vi "Align control label.vi"(8 "error in (no error)":errorcluster, 9 "label Position":T1, 11 "Ctl Refnum":refnum<vi>) -> (0 "error out":errorcluster, 3 "Ctl Refnum":refnum<vi>)   [LabVIEW 2009]
uses:
  label position.ctl
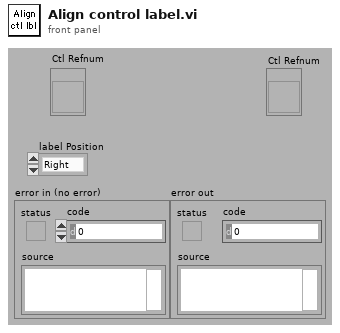
[diagram p1: front panel]
types:
  T1 = typedef "label position.ctl" = enum16{"Right", "Left", "Top left", "Top right"}
  T2 = typedef "LVPositionTypeDef.ctl" = cluster{"Left":i32, "Top":i32}
  T3 = typedef "LVBoundsTypeDef.ctl" = cluster{"Width":u32, "Height":u32}
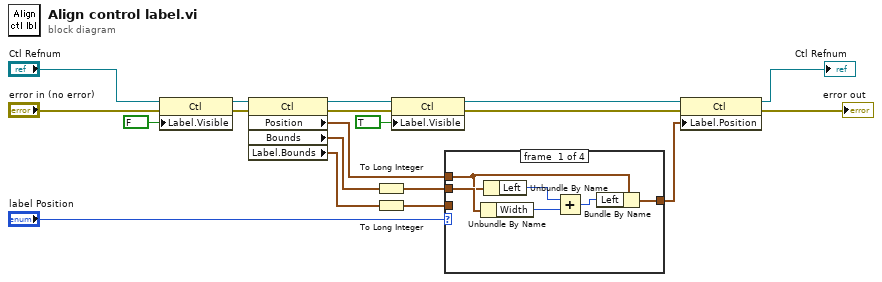
[diagram p0: block diagram]
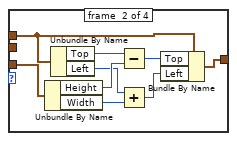
[diagram p2: hidden frame]
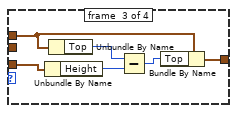
[diagram p3: hidden frame]
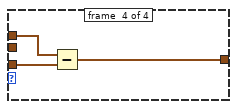
[diagram p4: hidden frame]
diagram:
  n1 = property class="Ctl"(reference="Ctl Refnum", error in="error in (no error)", "Label.Visible"=FALSE) -> (reference out=w9:refnum<vi>, error out=w7:errorcluster)
  n2 = property class="Ctl"(reference=w9, error in=w7) -> (reference out=w4:refnum<vi>, error out=w5:errorcluster, "Position"=w13:T2, "Bounds"=w14:T3, "Label.Bounds"=w18:T3)
  n3 = To Long Integer(number=w14) -> (32bit integer=w16:cluster{"Width":i32, "Height":i32})
  n4 = To Long Integer(number=w18) -> (32bit integer=w15:cluster{"Width":i32, "Height":i32})
  n5 = property class="Ctl"(reference=w4, error in=w5, "Label.Visible"=TRUE) -> (reference out=w1:refnum<vi>, error out=w2:errorcluster)
  n6 = case shown="\"Top right\"" "label Position" {
    tunnel: w16 -> [w25 _ _ _]
    tunnel: w13 -> [w23 w31 w37 w43]
    tunnel: w15 -> [_ w34 w40 w42]
    tunnel: [w22 w29 w35 w41] -> w17
    frame #0 {
      n7 = Unbundle By Name(w25) -> ("Width"=w20:i32)
      n8 = Unbundle By Name(w23) -> ("Left"=w24:i32)
      n9 = Add(x=w24, y=w20) -> (x+y=w21:i32)
      n10 = Bundle By Name(cluster=w23, "Left"=w21) -> (w22:T2)
    }
    frame #1 {
      n11 = Unbundle By Name(w34) -> ("Height"=w32:i32, "Width"=w28:i32)
      n12 = Unbundle By Name(w31) -> ("Top"=w33:i32, "Left"=w27:i32)
      n13 = Subtract(x=w33, y=w32) -> (x-y=w30:i32)
      n14 = Add(x=w27, y=w28) -> (x+y=w26:i32)
      n15 = Bundle By Name(cluster=w31, "Top"=w30, "Left"=w26) -> (w29:T2)
    }
    frame #2 {
      n16 = Unbundle By Name(w40) -> ("Height"=w38:i32)
      n17 = Unbundle By Name(w37) -> ("Top"=w39:i32)
      n18 = Subtract(x=w39, y=w38) -> (x-y=w36:i32)
      n19 = Bundle By Name(cluster=w37, "Top"=w36) -> (w35:T2)
    }
    frame #3 {
      n20 = Subtract(x=w43, y=w42) -> (x-y=w41:T2)
    }
  }
  n21 = property class="Ctl"(reference=w1, error in=w2, "Label.Position"=w17) -> (reference out=→"Ctl Refnum":refnum<vi>, error out=→"error out":errorcluster)
